vi "Set XY Graph Value.vi"   [LabVIEW 2016, in "graph_utilities.lvclass"]
uses:
  graph_utilities.lvclass
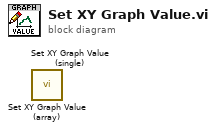
[diagram p0: block diagram]
diagram:
  n1 = call "Set XY Graph Value (array).vi"() -> ()  [unwired: 10 in, 2 out]
  n2 = call "Set XY Graph Value (single).vi"() -> ()  [unwired: 10 in, 2 out]
